vi "Start_Stop.vi"(9 "Enum":enum16{"Reset", "Abort"}(ring)=enum."Abort", 11 "Boolean in":bool=TRUE) -> (3 "Boolean out":bool)   [LabVIEW 2023, in "GUI.lvlib"]
uses:
  GUI.lvlib
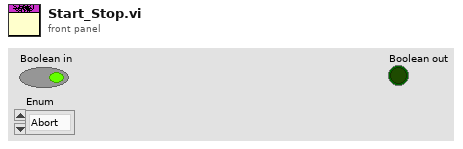
[diagram p1: front panel]
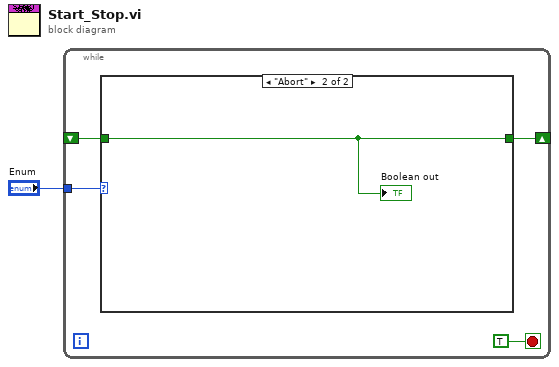
[diagram p0: block diagram]
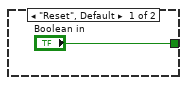
[diagram p2: hidden frame]
diagram:
  n1 = while {
    tunnel: "Enum" -> [w4]
    shift-right: [w3] -> _
    shift-left: _ -> [w2]
    stop <- TRUE stop-if-true
    n2 = case shown="\"Abort\"" w4 {
      tunnel: ["Boolean in" w7] -> w3
      tunnel: w2 -> [_ w7]
      frame "Reset", Default {
      }
      frame "Abort" {
        "Boolean out" <- w7
      }
    }
  }
